vi "Exit_Event_Handlervi.vi"(8 "error in (no error)":errorcluster, 10 "Exit?":bool=TRUE, 11 "Command":T1=enum."Generate Event") -> (0 "error out":errorcluster, 2 "Event Registration Refnum out":refnum<event-registration>, 3 "Exit":refnum<user-event>)   [LabVIEW 2021]
uses:
  Controls/Exit Event Handle Comamnd.ctl
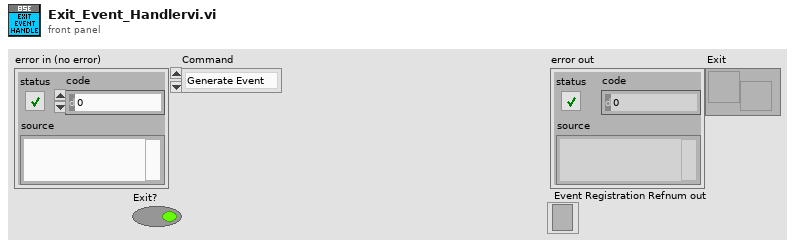
[diagram p1: front panel]
types:
  T1 = typedef "Exit Event Handle Comamnd.ctl" = enum16{"Init", "Close", "Generate Event"}
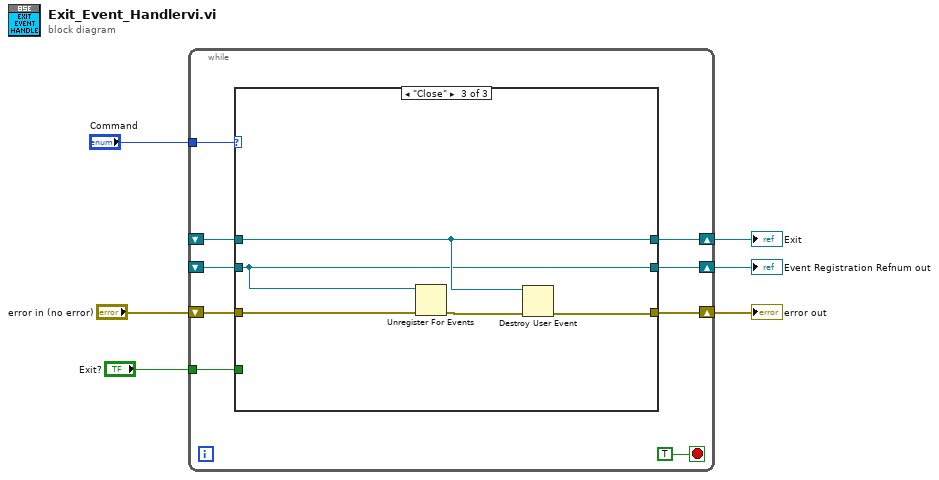
[diagram p0: block diagram]
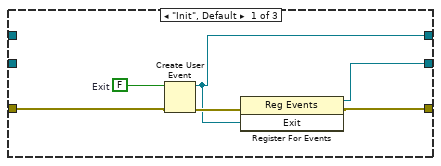
[diagram p2: hidden frame]
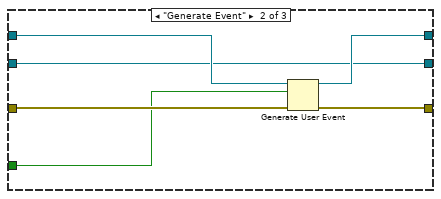
[diagram p3: hidden frame]
diagram:
  n1 = while {
    shift-right: [w15] -> w6
    shift-left: "error in (no error)" -> [w13]
    tunnel: "Command" -> [w11]
    shift-right: [w14] -> w5
    shift-left: _ -> [w10]
    shift-right: [w9] -> w2
    shift-left: _ -> [w8]
    tunnel: "Exit?" -> [w7]
    stop <- TRUE stop-if-true
    n2 = case shown="\"Close\"" w11 {
      tunnel: [w21 w26 w28] -> w15
      tunnel: [w20 w22 w29] -> w14
      tunnel: w13 -> [w17 w27 w31]
      tunnel: w10 -> [_ w22 w29]
      tunnel: [w16 w24 w30] -> w9
      tunnel: w8 -> [_ w25 w30]
      tunnel: w7 -> [_ w23 _]
      frame "Init", Default {
        w19 = FALSE  # Exit
        n3 = Create User Event(user event datatype=w19, error in=w17) -> (user event=w16:refnum<user-event>, error out=w18:errorcluster)
        n4 = register-events(error in=w18, w16) -> (reference out=w20:refnum<event-registration>, error out=w21:errorcluster)  [unwired: 1 in]
      }
      frame "Generate Event" {
        n5 = Generate User Event(user event=w25, event data cluster=w23, error in=w27) -> (user event out=w24:refnum<user-event>, error out=w26:errorcluster)  [unwired: 1 in]
      }
      frame "Close" {
        n6 = Unregister For Events(event registration refnum=w29, error in=w31) -> (error out=w32:errorcluster)
        n7 = Destroy User Event(user event=w30, error in=w32) -> (error out=w28:errorcluster)
      }
    }
  }
  "error out" <- w6
  "Event Registration Refnum out" <- w5
  "Exit" <- w2
